vi "VFP Alarming Enable Controls.vi"(0 "Name":refnum<vi> caption="名称", 1 "Limit":refnum<vi> caption="边界", 2 "Deadband":refnum<vi> caption="死区", 3 "Priority":refnum<vi> caption="优先级", 4 "ack mode":refnum<vi> caption="ack模式", 5 "Area":refnum<vi> caption="区域", 7 "Description":refnum<vi> caption="说明", 9 "Allow Logging":refnum<vi> caption="允许记录", 12 "Enable?":bool caption="启用？") -> ()   [LabVIEW 2016]
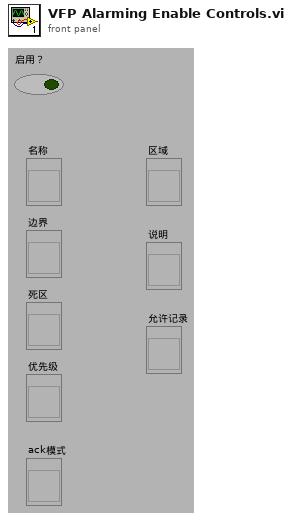
[diagram p1: front panel]
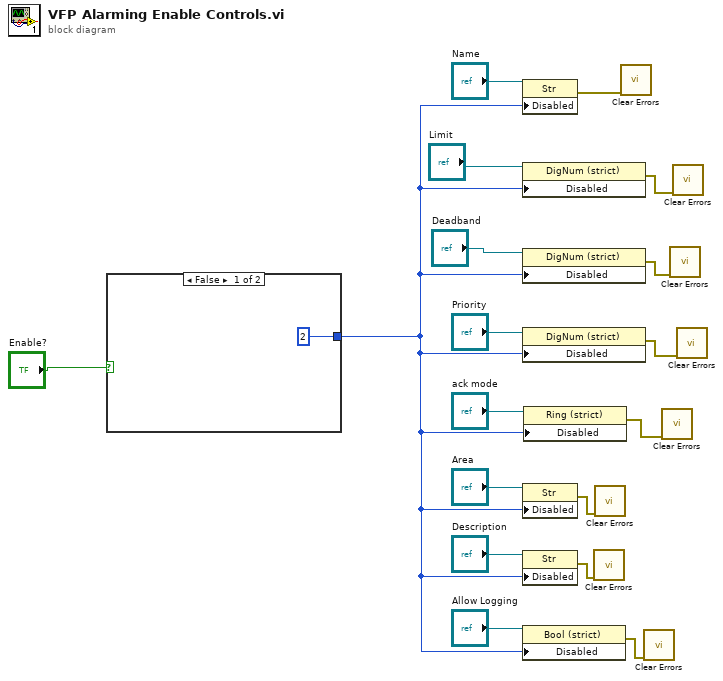
[diagram p0: block diagram]
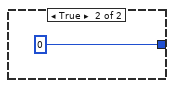
[diagram p2: hidden frame]
diagram:
  n1 = case shown="False" "Enable?" {
    tunnel: [2 0] -> w11
    frame False {
    }
    frame True {
    }
  }
  n2 = property class="Str"(reference="Name", "Disabled"=w11) -> (error out=w8:errorcluster)  [unwired: 1 in, 1 out]
  n3 = property class="DigNum (strict)"(reference="Limit", "Disabled"=w11) -> (error out=w7:errorcluster)  [unwired: 1 in, 1 out]
  n4 = property class="DigNum (strict)"(reference="Deadband", "Disabled"=w11) -> (error out=w6:errorcluster)  [unwired: 1 in, 1 out]
  n5 = property class="DigNum (strict)"(reference="Priority", "Disabled"=w11) -> (error out=w5:errorcluster)  [unwired: 1 in, 1 out]
  n6 = property class="Str"(reference="Area", "Disabled"=w11) -> (error out=w3:errorcluster)  [unwired: 1 in, 1 out]
  n7 = property class="Str"(reference="Description", "Disabled"=w11) -> (error out=w2:errorcluster)  [unwired: 1 in, 1 out]
  n8 = property class="Bool (strict)"(reference="Allow Logging", "Disabled"=w11) -> (error out=w1:errorcluster)  [unwired: 1 in, 1 out]
  n9 = property class="Ring (strict)"(reference="ack mode", "Disabled"=w11) -> (error out=w4:errorcluster)  [unwired: 1 in, 1 out]
  n10 = call <vilib>:"Clear Errors.vi"("error in (no error)"=w2) -> ()  [unwired: 5 in, 2 out]
  n11 = call <vilib>:"Clear Errors.vi"("error in (no error)"=w3) -> ()  [unwired: 5 in, 2 out]
  n12 = call <vilib>:"Clear Errors.vi"("error in (no error)"=w8) -> ()  [unwired: 5 in, 2 out]
  n13 = call <vilib>:"Clear Errors.vi"("error in (no error)"=w1) -> ()  [unwired: 5 in, 2 out]
  n14 = call <vilib>:"Clear Errors.vi"("error in (no error)"=w4) -> ()  [unwired: 5 in, 2 out]
  n15 = call <vilib>:"Clear Errors.vi"("error in (no error)"=w6) -> ()  [unwired: 5 in, 2 out]
  n16 = call <vilib>:"Clear Errors.vi"("error in (no error)"=w7) -> ()  [unwired: 5 in, 2 out]
  n17 = call <vilib>:"Clear Errors.vi"("error in (no error)"=w5) -> ()  [unwired: 5 in, 2 out]
